vi "Move Down Channel in Wfm Grp.vi"(7 "Channels Ctrl Ref":refnum<vi>, 8 "error in (no error)":errorcluster, 11 "To Save Wfm Arrays":waveform(dbl)[](array[waveform])) -> (0 "error out":errorcluster, 3 "Wfm Grp Data":T1)   [LabVIEW 2025, in "TDMS Waveform Creator UI.lvlib"]
uses:
  TDMS Waveform Creator UI.lvlib
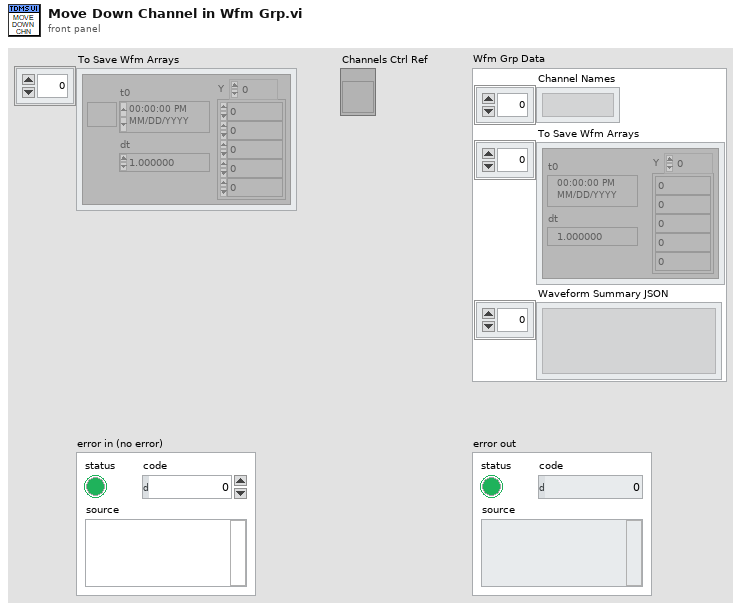
[diagram p1: front panel]
types:
  T1 = cluster{"Channel Names":string[], "To Save Wfm Arrays":waveform(dbl)[], "Waveform Summary JSON":string[]}
  T2 = cluster{"Item Names":string[], waveform(dbl)[], string[]}
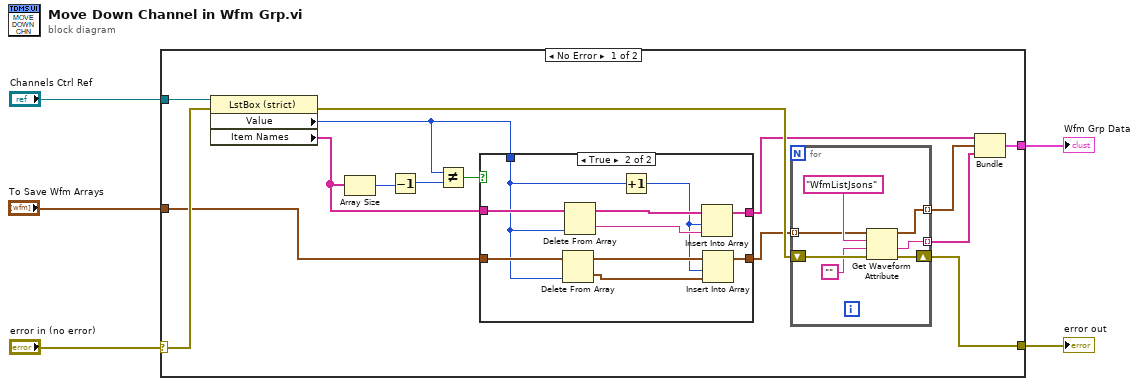
[diagram p0: block diagram]
diagram:
  n1 = case shown="No Error" "error in (no error)" {
    selector: "error in (no error)" -> [w19 w40]
    tunnel: "Channels Ctrl Ref" -> [w20 _]
    tunnel: "To Save Wfm Arrays" -> [w11 _]
    tunnel: [w17 w40] -> w2
    tunnel: [w14 _] -> w1
    frame No Error {
      n2 = property class="LstBox (strict)"(reference=w20, error in=w19) -> (error out=w18:errorcluster, "Value"=w13:i32, "Item Names"=w8:string[])  [unwired: 1 out]
      n3 = Array Size(array=w8) -> (size(s)=w7:i32)
      n4 = Decrement(x=w7) -> (x-1=w6:i32)
      n5 = Not Equal?(x=w13, y=w6) -> (x != y?=w12:bool)
      n6 = case shown="True" w12 {
        tunnel: w8 -> [w29 w39]
        tunnel: w11 -> [w28 w36]
        tunnel: w13 -> [_ w35]
        tunnel: [w29 w34] -> w9
        tunnel: [w28 w32] -> w10
        frame False {
        }
        frame True {
          n7 = Delete From Array(array=w36, index=w35) -> (deleted portion=w31:waveform(dbl), array with subset deleted=w38:waveform(dbl)[])  [unwired: 1 in]
          n8 = Delete From Array(array=w39, index=w35) -> (deleted portion=w33:string, array with subset deleted=w37:string[])  [unwired: 1 in]
          n9 = Increment(x=w35) -> (x+1=w30:i32)
          n10 = Insert Into Array(array=w37, index=w30, new element=w33) -> (w34:string[])
          n11 = Insert Into Array(array=w38, index=w30, new element=w31) -> (w32:waveform(dbl)[])
        }
      }
      n12 = for {
        shift-right: [w26] -> w17
        shift-left: w18 -> [w27]
        tunnel: [w25] -> w16 mode=indexing
        tunnel: [w22] -> w15 mode=indexing
        tunnel: w10 -> [w21] mode=indexing
        n13 = Get Waveform Attribute(4:w27, 5:"", 6:"WfmListJsons" ("name"), 7:w21) -> (0:w26:errorcluster, 1:w22:string, 3:w25:waveform(dbl))  [unwired: 1 out]
      }
      n14 = Bundle("Item Names"=w9, w16, w15) -> (w14:T2)  [unwired: 1 in]
    }
    frame Error {
    }
  }
  "error out" <- w2
  "Wfm Grp Data" <- w1
